vi "PQueue Add.vi"(10 "Path":T1, 11 "PQueue in":T1[](array[typedef])) -> (3 "PQueue out":T1[](array[typedef]))   [LabVIEW 2017]
uses:
  Path.ctl
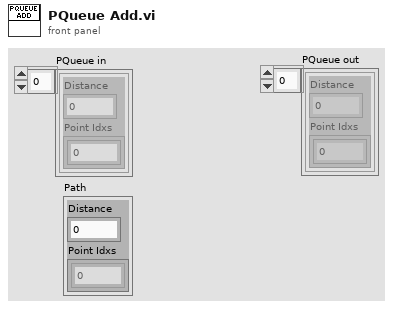
[diagram p1: front panel]
types:
  T1 = typedef "Path.ctl" = cluster{"Distance":dbl, "Point Idxs":i32[]}
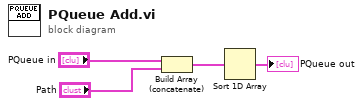
[diagram p0: block diagram]
diagram:
  n1 = Build Array (concatenate)("PQueue in", "Path") -> (w1:T1[])
  n2 = Sort 1D Array(array=w1) -> (sorted array=→"PQueue out":T1[])
